vi "motor_control_close_loop.vi"() -> ()   [LabVIEW 2014]
uses:
  <vilib>/Platform/TimedLoop/XDataNode/timing_clust.ctl
  <vilib>/Platform/TimedLoop/XDataNode/nitl_modes.ctl
  <vilib>/Platform/TimedLoop/XDataNode/wakeup.ctl
  <vilib>/myRIO/Common/Instrument Driver Framework/myRIO v1.0/Encoder/typedefs/Encoder Signal Mode.ctl
  <vilib>/myRIO/Instrument Drivers/Onboard IO/Encoder/typedefs/Encoder Reference.ctl
  <vilib>/myRIO/Common/Instrument Driver Framework/Utilities/typedefs/myRIO Generic Hardware Reference.ctl
  <vilib>/myRIO/Common/Instrument Driver Framework/Utilities/typedefs/Hardware Version Enum.ctl
  <vilib>/myRIO/Common/Instrument Driver Framework/Utilities/typedefs/myRIO v1.0 Reference.ctl
  <vilib>/myRIO/Common/Instrument Driver Framework/Utilities/typedefs/Generic FPGA Reference.ctl
  <vilib>/myRIO/Common/Instrument Driver Framework/myRIO v1.0/Encoder/typedefs/Encoder Channels Enum.ctl
  <vilib>/myRIO/Common/Instrument Driver Framework/myRIO v1.0/Encoder/typedefs/Encoder Configuration v1.0.ctl
  <vilib>/userdefined/High Color/nirio_resource_hc.ctl
  <vilib>/myRIO/Instrument Drivers/Onboard IO/PWM/typedefs/PWM Reference.ctl
  <vilib>/myRIO/Common/Instrument Driver Framework/myRIO v1.0/PWM/typedefs/PWM Channels Enum.ctl
  <vilib>/myRIO/Instrument Drivers/Onboard IO/PWM/typedefs/PWM Configuration.ctl
  <vilib>/myRIO/Common/Instrument Driver Framework/Utilities/vis/Is FPGA Ref Available.vi
  <vilib>/myRIO/Common/Instrument Driver Framework/myRIO v1.0/Encoder/vis/myRIO v1.1 Open Encoder.vi
  <vilib>/myRIO/Instrument Drivers/Onboard IO/Encoder/vis/Read.vi
  <vilib>/myRIO/Common/Instrument Driver Framework/myRIO v1.0/PWM/vis/myRIO v1.1 Open PWM.vi
  <vilib>/myRIO/Instrument Drivers/Onboard IO/PWM/vis/Set Duty Cycle and Frequency.vi
  <vilib>/myRIO/Instrument Drivers/Onboard IO/AI/vis/Read.vi
  <vilib>/myRIO/Common/Instrument Driver Framework/Utilities/vis/Validate Channels.vi
  <vilib>/myRIO/Common/Instrument Driver Framework/myRIO v1.0/Encoder/vis/myRIO v1.0 Reserve Encoder.vi
  <vilib>/myRIO/Instrument Drivers/Onboard IO/DIO/vis/Write.vi
  <vilib>/myRIO/Common/Instrument Driver Framework/myRIO v1.0/PWM/vis/myRIO v1.0 Reserve PWM.vi
  <vilib>/myRIO/Common/Instrument Driver Framework/myRIO v1.0/Encoder/vis/myRIO v1.0 Build MUX Configuration Encoder.vi
  <vilib>/myRIO/Common/Instrument Driver Framework/myRIO v1.0/Resource Manager/vis/myRIO v1.0 Reserve Channel List.vi
  <vilib>/myRIO/Common/Instrument Driver Framework/myRIO v1.0/PWM/vis/myRIO v1.0 Build MUX Configuration PWM.vi
  <vilib>/myRIO/Common/Instrument Driver Framework/myRIO v1.0/Resource Manager/vis/myRIO v1.0 Create Configuration List.vi
  <vilib>/myRIO/Common/Instrument Driver Framework/myRIO v1.0/Resource Manager/vis/myRIO v1.0 Reserve Channel.vi
  <vilib>/myRIO/Common/Instrument Driver Framework/myRIO v1.0/Resource Manager/vis/myRIO v1.0 Unreserve Channel.vi
  <vilib>/myRIO/Common/Instrument Driver Framework/myRIO v1.0/Resource Manager/vis/myRIO v1.0 Build Mutex Name.vi
  <vilib>/myRIO/Instrument Drivers/Onboard IO/AI/vis/Smart Open.vi
  <vilib>/Utility/error.llb/Error Cluster From Error Code.vi
  <vilib>/myRIO/Common/Instrument Driver Framework/myRIO v1.0/AI/vis/myRIO v1.0 Read AI.vi
  <vilib>/addons/control/pid/pid.llb/PID (DBL).vi
  <vilib>/Utility/VariantDataType/GetNumericInfo.vi
  <vilib>/myRIO/Common/Instrument Driver Framework/myRIO v1.0/myRIO v1.1 Open.vi
  <vilib>/myRIO/Common/Instrument Driver Framework/Utilities/vis/IO Manager.vi
  <vilib>/myRIO/Common/Instrument Driver Framework/Utilities/vis/Configuration Manager.vi
  <vilib>/myRIO/Common/Instrument Driver Framework/myRIO v1.0/Resource Manager/vis/myRIO v1.0 Configure IO.vi
  <vilib>/myRIO/Common/Instrument Driver Framework/myRIO v1.0/myRIO v1.0 Close.vi
  <vilib>/myRIO/Common/Instrument Driver Framework/myRIO v1.0/Encoder/vis/myRIO v1.0 Configure Encoder.vi
  <vilib>/myRIO/Common/Instrument Driver Framework/myRIO v1.0/Encoder/vis/myRIO v1.0 Read Encoder.vi
  <vilib>/myRIO/Instrument Drivers/Onboard IO/PWM/vis/Smart Open.vi
  <vilib>/myRIO/Common/Instrument Driver Framework/myRIO v1.0/PWM/vis/myRIO v1.0 Write PWM.vi
  <vilib>/myRIO/Instrument Drivers/Onboard IO/DIO/vis/Smart Open.vi
  <vilib>/myRIO/Common/Instrument Driver Framework/myRIO v1.0/DIO/vis/myRIO v1.0 Write DIO.vi
  <vilib>/platform/TimedLoop/XDataNode/XDataNode.xnode
  <vilib>/myRIO/Express VI/Onboard IO/Encoder/Encoder Express VI.xnode
  <vilib>/myRIO/Instrument Drivers/Onboard IO/Encoder/vis/myRIO Encoder Open.xnode
  <vilib>/myRIO/Express VI/Onboard IO/PWM/PWM Express VI.xnode
  <vilib>/myRIO/Instrument Drivers/Onboard IO/PWM/vis/myRIO PWM Open.xnode
  <vilib>/Platform/TimedLoop/XDataNode/XDNodeRunTimeDep.lvlib
  <vilib>/myRIO/Instrument Drivers/Onboard IO/PWM/PWM.lvlib
  <vilib>/myRIO/Instrument Drivers/Onboard IO/Encoder/Encoder.lvlib
  <vilib>/addons/control/pid/NI_PID_pid.lvlib
  <vilib>/ptbypt/NI_PtbyPt.lvlib
panel:
  out "V_In":dbl
  in  "reinitialize? (F)":bool
  out "Angluar_average":dbl
  out "Angluar Rate_average":dbl
  out "Angluar Rate":dbl
  out "Angle_org":dbl(graph)
  in  "initialize_org":bool
  out "Angle_average":dbl(graph)
  in  "initialize_average":bool
  out "Angluar Rate_average":dbl(graph)
  out "Angluar Rate 2":dbl(graph)
  out "position_B":i32
  in  "Reset_B":bool
  out "velocity_B":dbl(graph)
  out "velocity_A":dbl(graph)
  in  "Reset_A":bool
  out "position_A":i32
  in  "电机开关":bool
  in  "关闭程序":bool
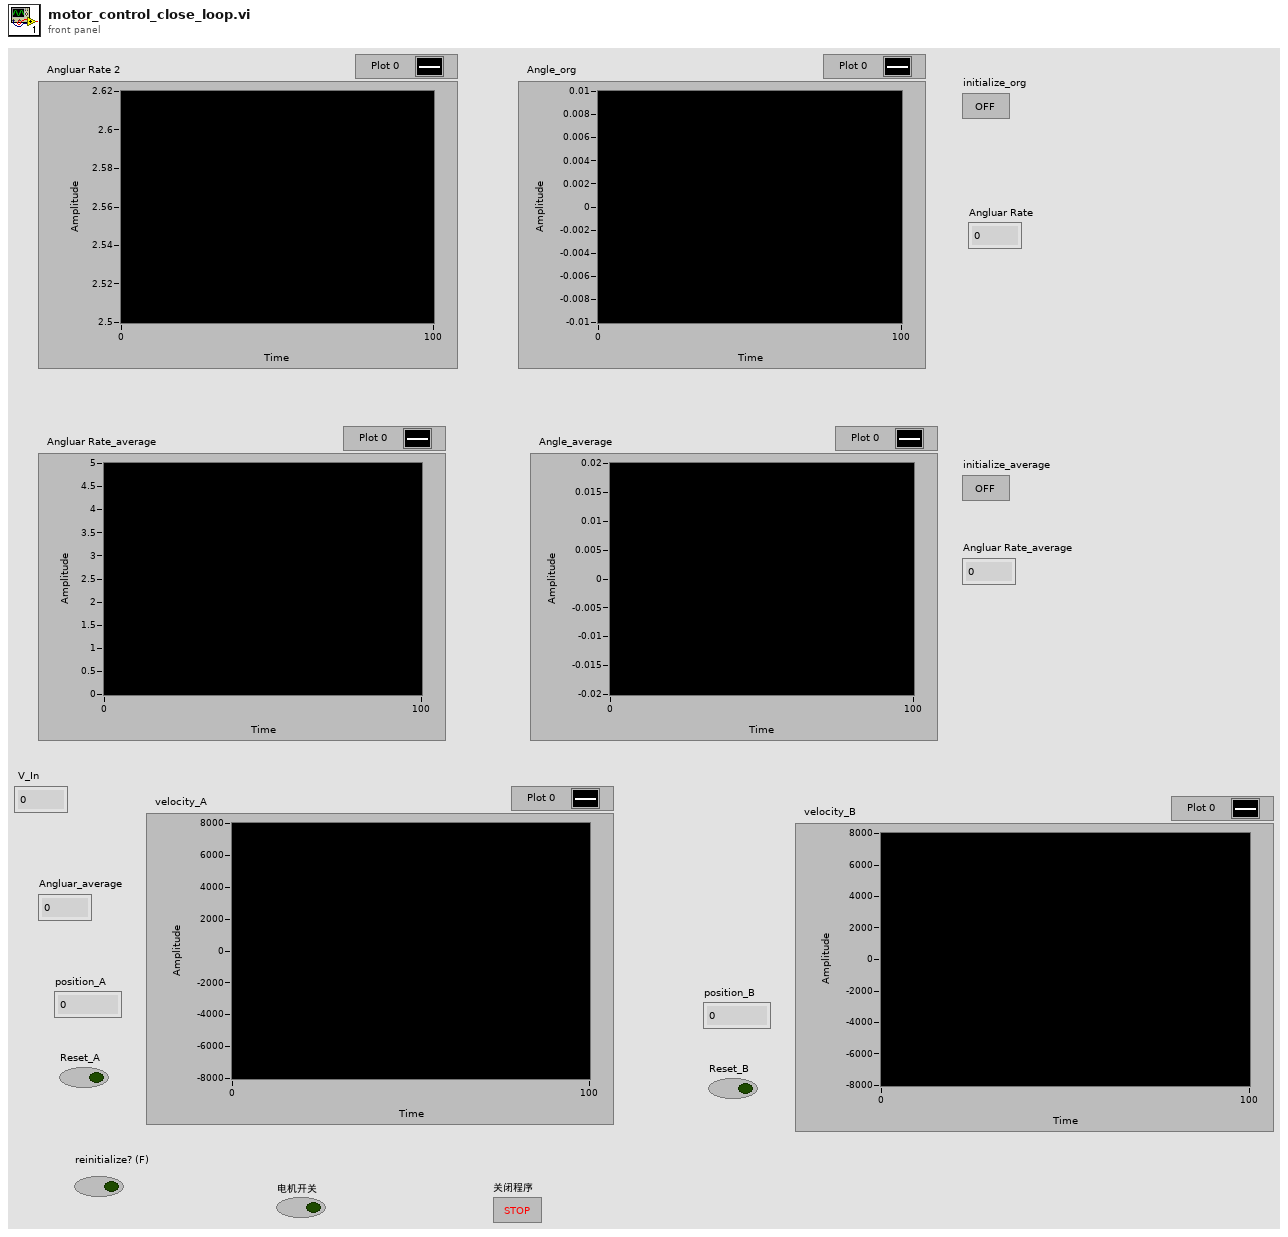
[diagram p1: front panel]
types:
  T1 = typedef "XDNodeRunTimeDep.lvlib/timing_clust.ctl" = cluster{"Expected End [f-1]":u64, "Actual End [f-1]":u64, "Finished Late? [f-1]":bool, "Expected End [i-1]":u64, "Actual End [i-1]":u64, "Finished Late? [i-1]":bool, "Expected Start [i]":u64, "Actual Start [i]":u64, "Expected Start [f]":u64, "Actual Start [f]":u64, "Source Name":string, "Structure Name":string, "Period":i64, "Deadline":i64, "Offset":i64, "Start":i64, "Priority":i32, "Timeout":i32, "Mode":T2, "Wakeup Reason":T3, "Error":errorcluster, "Source Type":string, "Secondary Source Type":string, "Global End Time":u64, "Global Start Time":u64, "Frame Duration":u64, "Iteration Duration":u64, "Assigned CPU":i32, "I/O Scan Engine Mode":u32}
  T2 = typedef "XDNodeRunTimeDep.lvlib/nitl_modes.ctl" = enum32{"No Change", "Process missed periods, maintain original phase", "Discard missed periods, maintain original phase", "Process missed periods, ignore original phase", "Discard missed periods, ignore original phase"}
  T3 = typedef "XDNodeRunTimeDep.lvlib/wakeup.ctl" = enum32{"Normal", "Aborted", "Asynchronous wakeup", "Timing source error", "Timed loop error", "Timeout"}
  T4 = cluster{"proportional gain (Kc)":dbl, "integral time (Ti, min)":dbl, "derivative time (Td, min)":dbl}
  T5 = typedef "Encoder.lvlib/Encoder Reference.ctl" = cluster{"myRIO Reference":T6, "Encoder Channels Enum":T10}
  T6 = typedef "myRIO Generic Hardware Reference.ctl" = cluster{"myRIO Model":T7, "myRIO Hardware Reference":T8}
  T7 = typedef "Hardware Version Enum.ctl" = enum16{"Unknown", "myRIO-1900", "myRIO-1950"}
  T8 = typedef "myRIO v1.0 Reference.ctl" = cluster{"Generic FPGA Reference":T9, "Allow multiple opens":bool}
  T9 = typedef "Generic FPGA Reference.ctl" = refnum<k20>
  T10 = typedef "Encoder Channels Enum.ctl" = enum16{"Not Connected", "C/ENC0", "C/ENC1", "A/ENC", "B/ENC"}
  T11 = typedef "Encoder Signal Mode.ctl" = enum16{"Quadrature phase signal", "Step and direction signal"}
  T12 = typedef "nirio_resource_hc.ctl" = tag
  T13 = typedef "PWM.lvlib/PWM Reference.ctl" = cluster{"myRIO Reference":T6, "PWM Channels Enum":T14, "PWM Configuration":T15}
  T14 = typedef "PWM Channels Enum.ctl" = enum16{"Not Connected", "C/PWM0", "C/PWM1", "A/PWM0", "A/PWM1", "A/PWM2", "B/PWM0", "B/PWM1", "B/PWM2"}
  T15 = typedef "PWM.lvlib/PWM Configuration.ctl" = cluster{"Frequency":dbl, "Duty Cycle":dbl}
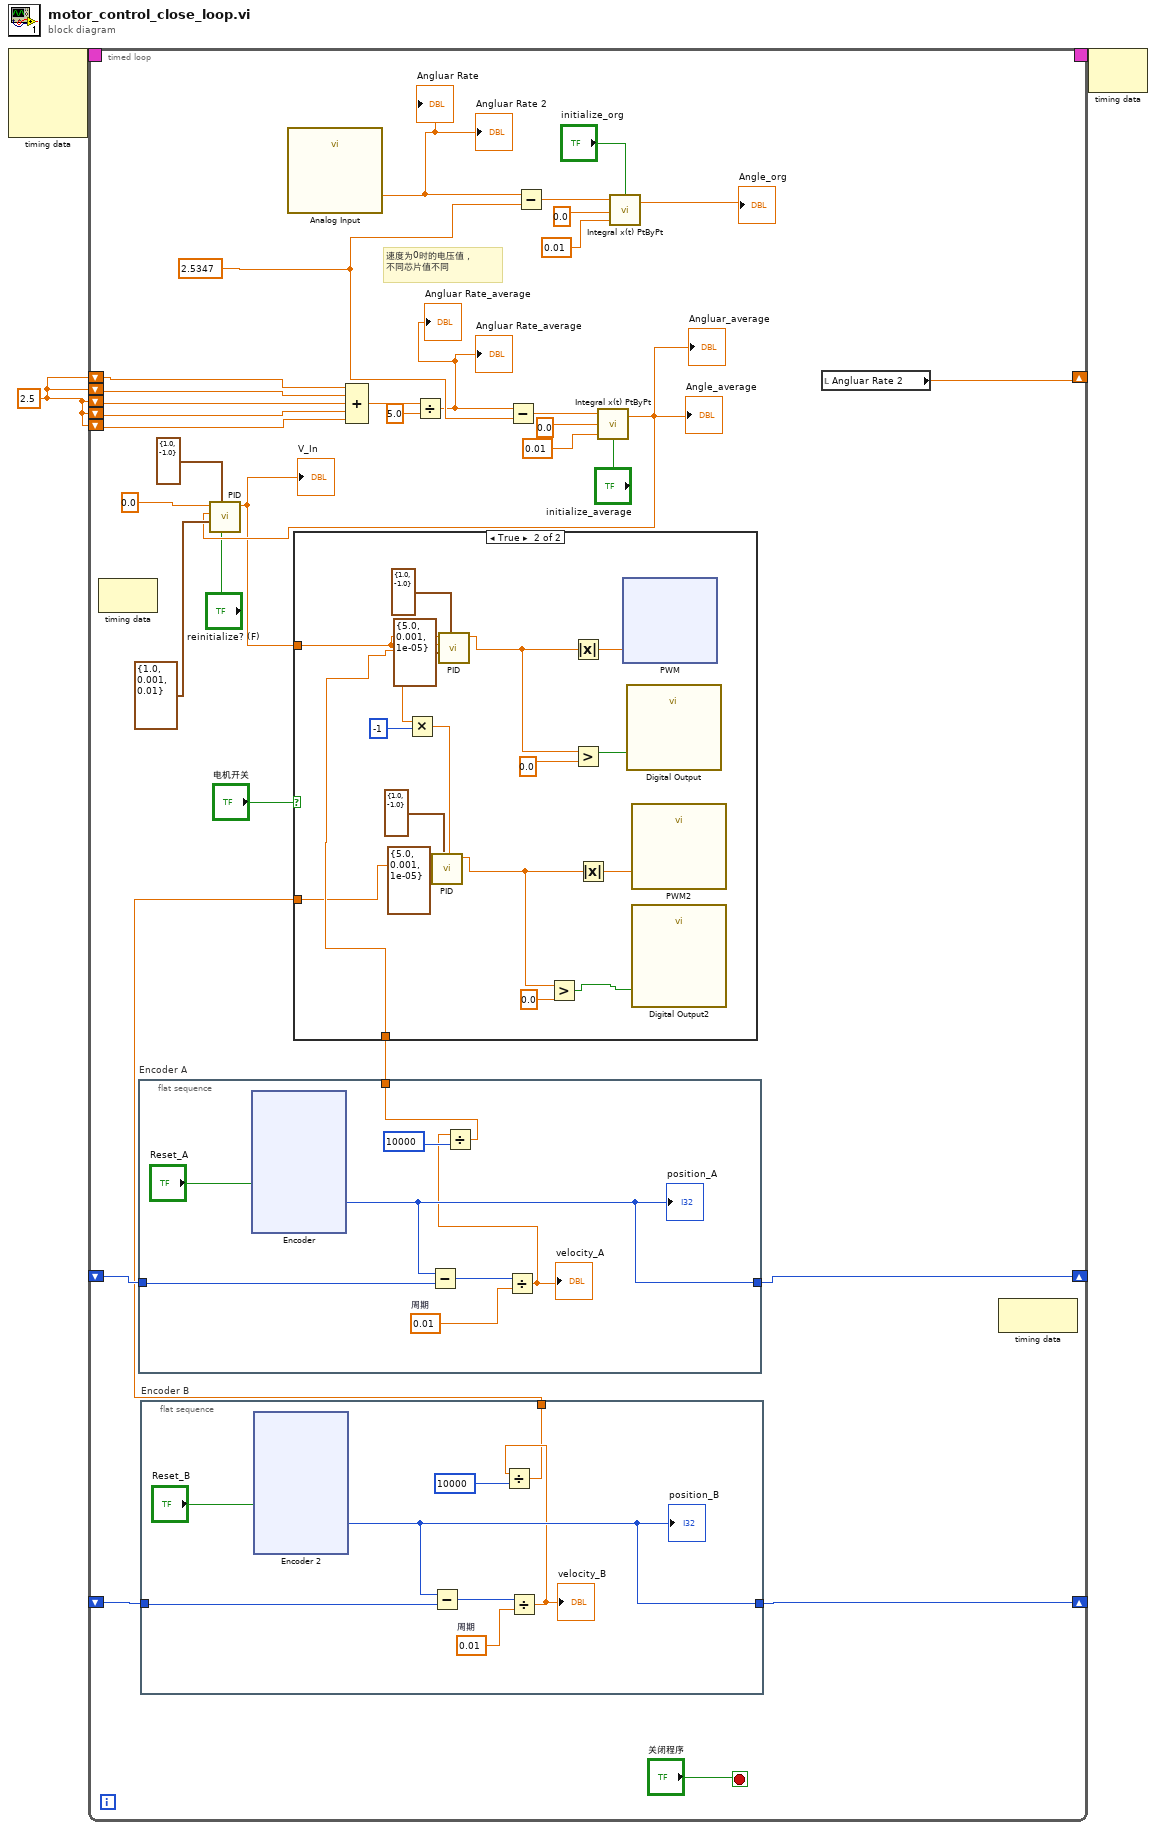
[diagram p0: block diagram]
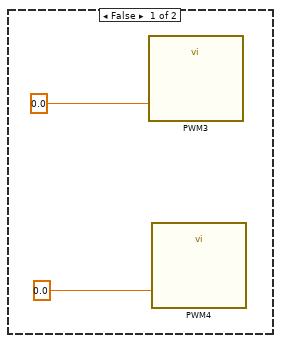
[diagram p2: hidden frame]
diagram:
  w1 = 2.5
  n1 = node-c288() -> (w3:T1)  [unwired: 4 in]
  n2 = timed-loop {
    timing: w3 -> [_]
    timing-out: [_] -> w2
    shift-right: [w35] -> _
    shift-left: _ -> [w34]
    shift-right: [w32] -> _
    shift-left: _ -> [w33]
    shift-right: [w16] -> _
    shift-left: w1 -> [w15]
    shift-left: w1 -> [w14]
    shift-left: w1 -> [w13]
    shift-left: w1 -> [w12]
    shift-left: w1 -> [w11]
    stop <- "关闭程序" stop-if-true
    w17 = 2.5347
    # "速度为0时的电压值，\n不同芯片值不同"
    n3 = node-c288() -> ()  [unwired: 1 in, 1 out]
    n4 = flat-sequence "Encoder A" {
      tunnel: [w98] -> w35
      tunnel: w34 -> [w97]
      tunnel: [w93] -> w31
      frame #0 {
        w95 = 0.01  # 周期
        n5 = xnode "Encoder"("Reset Counter"="Reset_A") -> ("Counter Value"=w98:i32)  [unwired: 1 in, 3 out]
        "position_A" <- w98
        n6 = Subtract(x=w98, y=w97) -> (x-y=w96:i32)
        n7 = Divide(x=w96, y=w95) -> (x/y=w92:dbl)
        "velocity_A" <- w92
        n8 = Divide(x=w92, y=10000) -> (x/y=w93:dbl)
      }
    }
    n9 = flat-sequence "Encoder B" {
      tunnel: [w44] -> w32
      tunnel: w33 -> [w43]
      tunnel: [w38] -> w30
      frame #0 {
        w41 = 0.01  # 周期
        n10 = xnode "Encoder 2"("Reset Counter"="Reset_B") -> ("Counter Value"=w44:i32)  [unwired: 1 in, 3 out]
        "position_B" <- w44
        n11 = Subtract(x=w44, y=w43) -> (x-y=w42:i32)
        n12 = Divide(x=w42, y=w41) -> (x/y=w39:dbl)
        "velocity_B" <- w39
        n13 = Divide(x=w39, y=10000) -> (x/y=w38:dbl)
      }
    }
    n14 = call "Analog Input"() -> ("B/AI0 (Pin 3)"=w20:dbl)  [unwired: 26 in, 1 out]
    "Angluar Rate 2" <- w20
    "Angluar Rate" <- w20
    n15 = Compound Arithmetic op=ADD(w15, w14, w13, w12, w11) -> (w29:dbl)
    n16 = Divide(x=w29, y=5.0) -> (x/y=w10:dbl)
    "Angluar Rate_average" <- w10
    "Angluar Rate_average" <- w10
    n17 = Subtract(x=w10, y=w17) -> (x-y=w27:dbl)
    n18 = Subtract(x=w20, y=w17) -> (x-y=w23:dbl)
    n19 = call <vilib>:"Integral x(t) PtByPt.vi"("initialize"="initialize_average", "dt"=0.01, "initial condition"=0.0, "x"=w27) -> ("integral x(t)"=w6:dbl)  [unwired: 1 out]
    "Angle_average" <- w6
    "Angluar_average" <- w6
    n20 = call-poly <vilib>:"PID.vi"("reinitialize? (F)"="reinitialize? (F)", "output range"=cluster{"output high":dbl, "output low":dbl} {"output high"=1.0, "output low"=-1.0}, "PID gains"=T4 {"proportional gain (Kc)"=1.0, "integral time (Ti, min)"=0.001, "derivative time (Td, min)"=0.01}, "process variable"=w6, "setpoint"=0.0) -> ("output"=w4:dbl)  [unwired: 5 in, 1 out]
    "V_In" <- w4
    n21 = case shown="True" "电机开关" {
      tunnel: w31 -> [_ w159]
      tunnel: w30 -> [_ w157]
      tunnel: w4 -> [_ w150]
      frame False {
        n22 = call "PWM3"("Duty Cycle (0-1)"=0.0) -> ()  [unwired: 26 in, 1 out]
        n23 = call "PWM4"("Duty Cycle (0-1)"=0.0) -> ()  [unwired: 26 in, 1 out]
      }
      frame True {
        n24 = Multiply(x=w150, y=-1) -> (x*y=w154:dbl)
        n25 = call-poly <vilib>:"PID.vi"("output range"=cluster{"output high":dbl, "output low":dbl} {"output high"=1.0, "output low"=-1.0}, "PID gains"=T4 {"proportional gain (Kc)"=5.0, "integral time (Ti, min)"=0.001, "derivative time (Td, min)"=1e-05}, "process variable"=w157, "setpoint"=w154) -> ("output"=w158:dbl)  [unwired: 6 in, 1 out]
        n26 = call-poly <vilib>:"PID.vi"("output range"=cluster{"output high":dbl, "output low":dbl} {"output high"=1.0, "output low"=-1.0}, "PID gains"=T4 {"proportional gain (Kc)"=5.0, "integral time (Ti, min)"=0.001, "derivative time (Td, min)"=1e-05}, "process variable"=w159, "setpoint"=w150) -> ("output"=w160:dbl)  [unwired: 6 in, 1 out]
        n27 = Greater?(x=w158, y=0.0) -> (0:w153:bool)
        n28 = Absolute Value(x=w160) -> (abs(x)=w163:dbl)
        n29 = Greater?(x=w160, y=0.0) -> (0:w156:bool)
        n30 = Absolute Value(x=w158) -> (abs(x)=w161:dbl)
        n31 = xnode "PWM"("Duty Cycle"=w163) -> ()  [unwired: 1 in, 1 out]
        n32 = call "Digital Output"("A/DIO0 (Pin 11)"=w156) -> ()  [unwired: 26 in, 1 out]
        n33 = call "PWM2"("Duty Cycle (0-1)"=w161) -> ()  [unwired: 26 in, 1 out]
        n34 = call "Digital Output2"("B/DIO0 (Pin 11)"=w153) -> ()  [unwired: 26 in, 1 out]
      }
    }
    n35 = call <vilib>:"Integral x(t) PtByPt.vi"("initialize"="initialize_org", "dt"=0.01, "initial condition"=0.0, "x"=w23) -> ("integral x(t)"=→"Angle_org":dbl)  [unwired: 1 out]
    n36 = local read "Angluar Rate 2"() -> (w16:dbl)
    n37 = node-c288() -> ()  [unwired: 1 in, 1 out]
  }
  n38 = node-c288(w2) -> ()  [unwired: 1 out]
